vi "Read RawData.vi"(8 "error in (no error)":errorcluster, 9 "WCM_max_value":bool, 10 "# of scans":i32, 11 "UV-VIS-Avantes in":refnum<class "UV-VIS-Avantes.lvclass">) -> (0 "error out":errorcluster, 1 "Channel II":i32[][](array[numeric]), 2 "Channel I":i32[][](array[numeric]), 3 "UV-VIS-Avantes out":refnum<class "UV-VIS-Avantes.lvclass">, 4 "WCM_values":sgl[](array[numeric]))   [LabVIEW 2015, in "UV-VIS-Avantes.lvclass"]
uses:
  UV-VIS-Avantes.lvclass
  Detector.lvclass
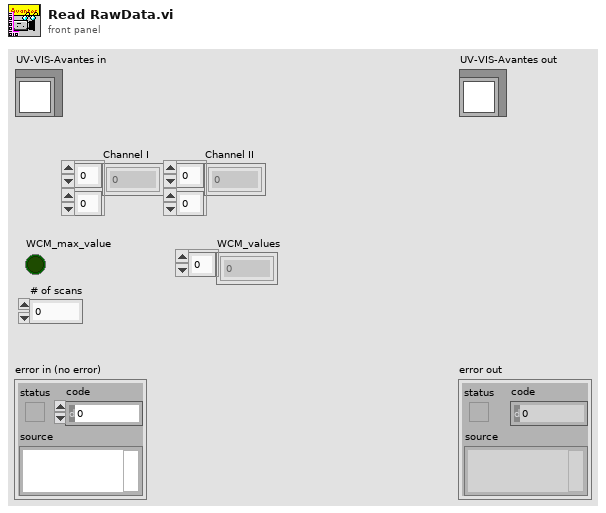
[diagram p1: front panel]
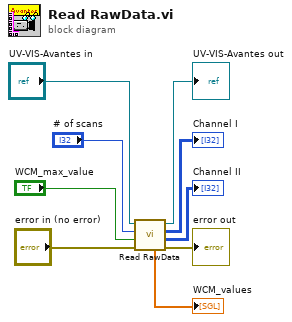
[diagram p0: block diagram]
diagram:
  n1 = call-parent "Read RawData.vi"("error in (no error)"="error in (no error)", "WCM_max_value"="WCM_max_value", "# of scans"="# of scans", "Detector in"="UV-VIS-Avantes in") -> ("error out"=→"error out":errorcluster, "Channel II"=→"Channel II":i32[][], "Channel I"=→"Channel I":i32[][], "Detector out"=→"UV-VIS-Avantes out":refnum<class "UV-VIS-Avantes.lvclass">, "WCM_values"=→"WCM_values":sgl[])  [unwired: 3 in]
